vi "Configuration2.vi"() -> ()   [LabVIEW 2016]
uses:
  <vilib>/MakerHub/LINX/Public/Peripherals/Digital/Digital Write 1 Chan.vi
  <vilib>/MakerHub/LINX/Public/Peripherals/Digital/Digital Write N Chans.vi
  <vilib>/MakerHub/LINX/Private/Local IO/LinxDigitalWrite.vi
  <vilib>/MakerHub/LINX/Public/Utilities/Check Channel.vi
  <vilib>/MakerHub/LINX/Public/Utilities/Open Serial.vi
  <vilib>/MakerHub/LINX/Private/Utilties/Generate Error.vi
  <vilib>/MakerHub/LINX/LMH-LINX.lvlib
panel:
  in  "Serial Port":refnum<visa-resource-name>="COM5"
  in  "I- Pin#":u8=45
  in  "I+ Pin#":u8=31
  in  "V- Pin#":u8=39
  in  "V+ Pin#":u8=37
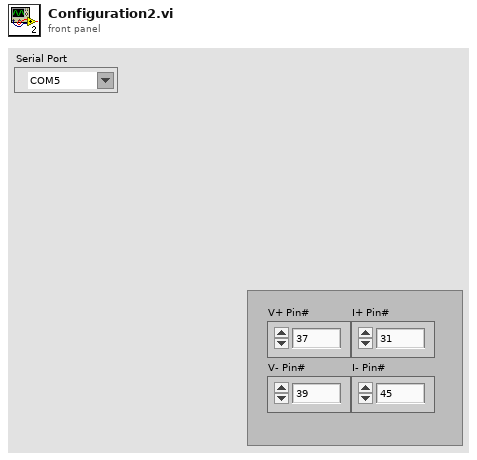
[diagram p1: front panel]
types:
  T1 = typedef "LMH-LINX.lvlib/LINX Ref.ctl" = cluster{"IO":T2, "Interface":T3, "LINX Device Config":T4}
  T2 = typedef "LMH-LINX.lvlib/Platform.ctl" = enum16{"Remote", "Local"}
  T3 = typedef "LMH-LINX.lvlib/Interface.ctl" = enum16{"Serial", "TCP"}
  T4 = typedef "LMH-LINX.lvlib/Device.lvlib/LINX Device Config.ctl" = cluster{"Interface":T3, "COM Port":refnum<visa-resource-name>, "TCP Configuration":T5, "Device Family":u8, "Device ID":u8, "Device Name":string, "TCP Ref":refnum<k5>, "Channels":T6}
  T5 = typedef "LMH-LINX.lvlib/Device.lvlib/TCP Config.ctl" = cluster{"IP Address":string, "Port":u16}
  T6 = typedef "LMH-LINX.lvlib/Channels.ctl" = cluster{"DI":u8[], "DO":u8[], "AI":u8[], "AO":u8[], "PWM":u8[], "QE":u8[], "UART":u8[], "I2C 2":u8[], "SPI":u8[], "CAN":u8[], "Servo":u8[], "AI Ref (V)":dbl, "AI Resolution (Bits)":u8, "AO Ref (V)":dbl, "AO Resolution (Bits)":u8}
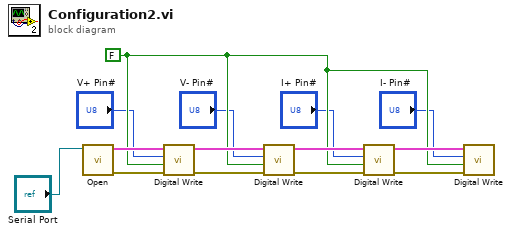
[diagram p0: block diagram]
diagram:
  w5 = FALSE
  n1 = call-poly <vilib>:"Open.vi"("Serial Port"="Serial Port") -> ("Error Out"=w12:errorcluster, "LINX Resource"=w13:T1)  [unwired: 8 in, 1 out]
  n2 = call-poly <vilib>:"Digital Write.vi"("Error In"=w12, "Output Value"=w5, "DO Channel"="V+ Pin#", "LINX Resource"=w13) -> ("Error Out"=w11:errorcluster, "LINX Resource"=w10:T1)  [unwired: 6 in]
  n3 = call-poly <vilib>:"Digital Write.vi"("Error In"=w11, "Output Value"=w5, "DO Channel"="V- Pin#", "LINX Resource"=w10) -> ("Error Out"=w9:errorcluster, "LINX Resource"=w8:T1)  [unwired: 6 in]
  n4 = call-poly <vilib>:"Digital Write.vi"("Error In"=w9, "Output Value"=w5, "DO Channel"="I+ Pin#", "LINX Resource"=w8) -> ("Error Out"=w6:errorcluster, "LINX Resource"=w7:T1)  [unwired: 6 in]
  n5 = call-poly <vilib>:"Digital Write.vi"("Error In"=w6, "Output Value"=w5, "DO Channel"="I- Pin#", "LINX Resource"=w7) -> ()  [unwired: 6 in, 2 out]
